vi "Load IOPanel.vi"(8 "error in (no error)":errorcluster, 11 "MPC_VirbVision in":refnum<class "MPC_VirbVision.lvclass">) -> (0 "error out":errorcluster, 2 "This VI":refnum<vi>, 3 "MPC_VirbVision out":refnum<class "MPC_VirbVision.lvclass">)   [LabVIEW 2019, in "MPC_VirbVision.lvclass"]
uses:
  MPC_VirbVision.lvclass
  <vilib>/Utility/miscctls.llb/LVPositionTypeDef.ctl
  Function/IO Folder/IO_Class/IOCard.lvclass
  Function/IO Folder/IO_VI/IOCtrl/Ctrl/IO Card_Type.ctl
  Function/IO Folder/IO_Class/IOCard.lvclass/IOCard.ctl
panel:
  in  "Tab Control":enum32{"Page 1", "Page 2"}(tab)
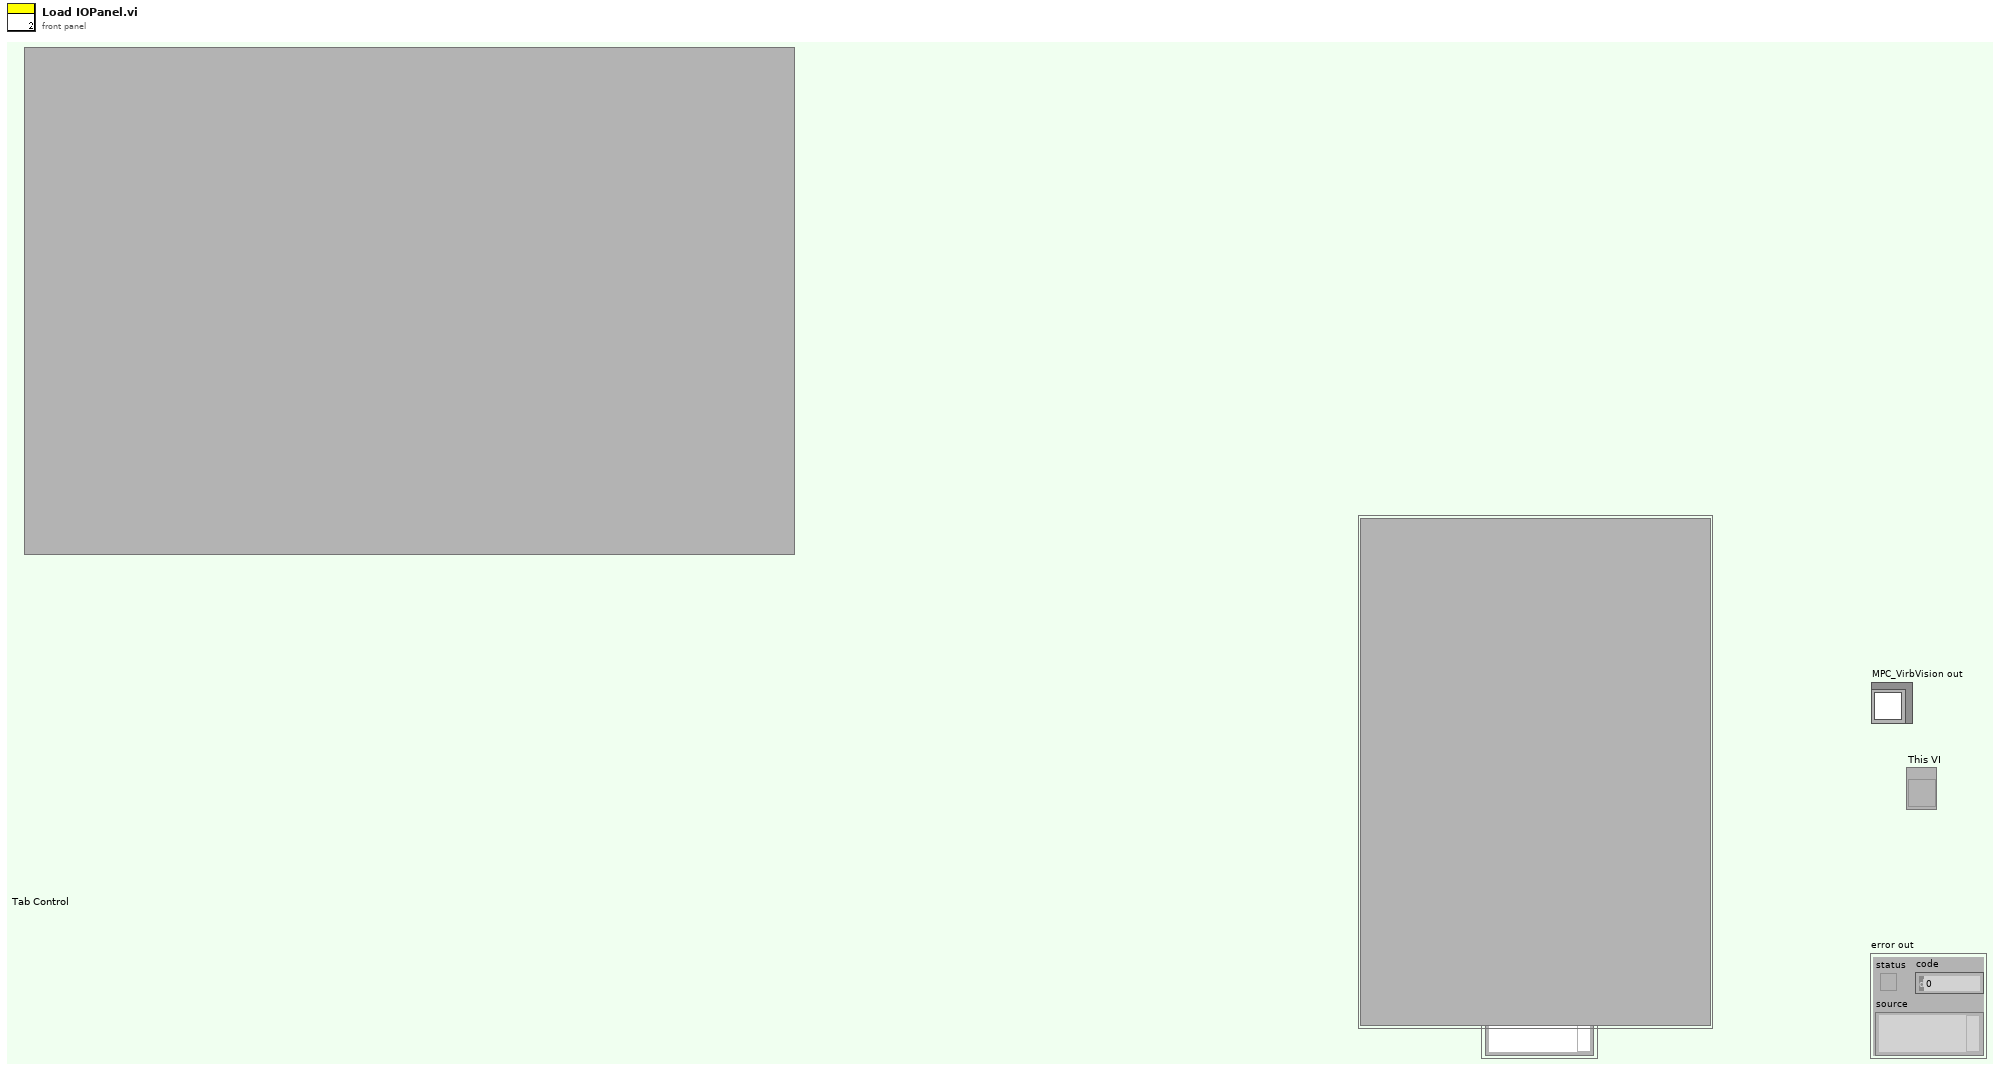
[diagram p1: front panel]
types:
  T1 = typedef "LVPositionTypeDef.ctl" = cluster{"Left":i32, "Top":i32}
  T2 = typedef "IO Card_Type.ctl" = enum16{"None", "Unidaq32", "6480", "2410C-64", "Zan", "DMC1000B", "16InOut", "Robot", "DMC3600"}
  T3 = cluster{"IO Card Type":T2, "IOType":enum16{"Input", "Output"}, "CardNumber":i32, "ConnectAct":bool, "IP":string}
  T4 = typedef "LVPointTypeDef.ctl" = cluster{"Horizontal":i16, "Vertical":i16}
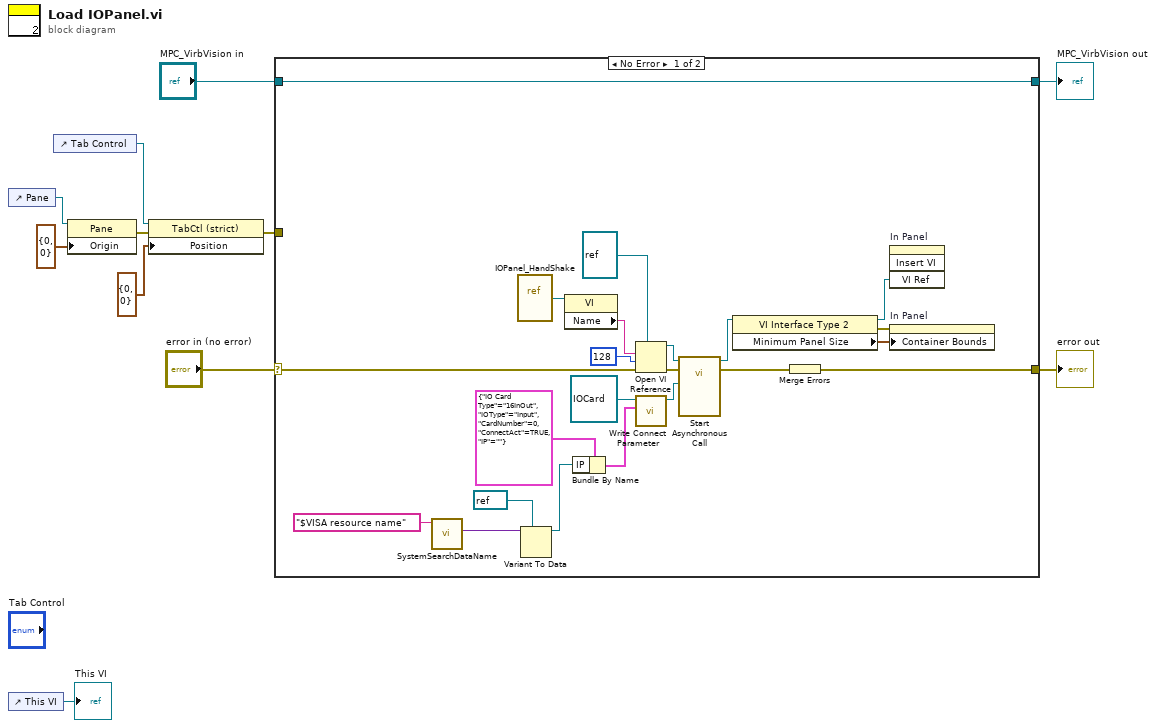
[diagram p0: block diagram]
diagram:
  n1 = control-ref of="Pane"() -> (w3:refnum<vi>)
  n2 = control-ref of="This VI"() -> (→"This VI":refnum<vi>)
  n3 = control-ref of="Tab Control"() -> (w2:refnum<vi>)
  n4 = property class="Pane"(reference=w3, "Origin"=T1 {"Left"=0, "Top"=0} ("Position")) -> (error out=w6:errorcluster)  [unwired: 1 in, 1 out]
  n5 = property on="Property Node" class="TabCtl (strict)"(reference=w2, error in=w6, "Position"=T1 {"Left"=0, "Top"=0}) -> (error out=w4:errorcluster)  [unwired: 1 out]
  n6 = case shown="No Error" "error in (no error)" {
    selector: "error in (no error)" -> [w30 w34]
    tunnel: [w22 w34] -> w8
    tunnel: [w25 w35] -> w11
    tunnel: "MPC_VirbVision in" -> [w25 w35]
    tunnel: w4 -> [_ _]
    frame No Error {
      n7 = call "SystemSearchDataName.vi"("element"="$VISA resource name") -> ("variant"=w15:variant)  [unwired: 8 in, 2 out]
      n8 = vi-ref "IOPanel_HandShake.vi"() -> (w33:refnum<vi>)
      n9 = Variant To Data(type=refnum<visa-resource-name> refnum ("VISA resource name"), Variant=w15) -> (data=w12:refnum<visa-resource-name>)  [unwired: 1 in, 1 out]
      n10 = property class="VI"(reference=w33) -> ("Name"=w32:string)  [unwired: 1 in, 2 out]
      n11 = Bundle By Name(cluster=T3 {"IO Card Type"=enum."16InOut", "IOType"=enum."Input", "CardNumber"=0, "ConnectAct"=TRUE, "IP"=""} ("Connect Parameter"), "IP"=w12) -> (w16:T3)
      n12 = Open VI Reference(type specifier VI Refnum (for type only)=refnum<vi> refnum, vi path=w32, options=128, error in (no error)=w30) -> (vi reference=w26:refnum<vi>, error out=w29:errorcluster)  [unwired: 2 in]
      n13 = call "Write Connect Parameter.vi"("Connect Parameter"=w16, "IOCard in"=refnum<class "IOCard.lvclass"> refnum ("IOCard In")) -> ("IOCard out"=w23:refnum<class "IOCard.lvclass">)  [unwired: 8 in, 1 out]
      n14 = call-by-ref "Start Asynchronous Call"(reference=w26, error in=w29, "IOCard In"=w23) -> (reference out=w20:refnum<vi>, error out=w28:errorcluster)  [unwired: 11 in]
      n15 = property class="VI Interface Type 2"(reference=w20) -> (reference out=w19:refnum<vi>, error out=w18:errorcluster, "Minimum Panel Size"=w21:T4)  [unwired: 1 in]
      n16 = Merge Errors(w28) -> (w22:errorcluster)
      n17 = invoke on="In Panel" class="SubPnl" method="Insert VI"("VI Ref"=w19) -> ()  [unwired: 3 in, 4 out]
      n18 = property on="In Panel" class="SubPnl"(error in=w18, "Container Bounds"=w21) -> ()  [unwired: 1 in, 2 out]
    }
    frame Error {
    }
  }
  "error out" <- w8
  "MPC_VirbVision out" <- w11
